vi "Get Speed For Shooting.vi"() -> (3 "Speed":dbl)   [LabVIEW 2016]
uses:
  Shared/Shooter Speed Type Def.ctl
  <vilib>/Rock Robotics/Network Tables/NT Read Boolean.vi
  Implementation/Ball Shooter Global.vi
  Framework/Robot Global Data.vi
  <vilib>/Analysis/NI_AALPro.lvlib
panel:
  in  "ClockWork":T1[](array[typedef])=[{"Distance"=8.5, "Speed"=5.4}, {"Distance"=10.9, "Speed"=6.3}, {"Distance"=8.1, "Speed"=5.1}]
  in  "Debug":bool
  out "XY Graph":cluster{dbl[], dbl[]}[](graph)
  in  "Veronica":T1[](array[typedef])=[{"Distance"=4.5, "Speed"=4.5}, {"Distance"=6.0, "Speed"=5.5}, {"Distance"=5.7, "Speed"=5.1}]
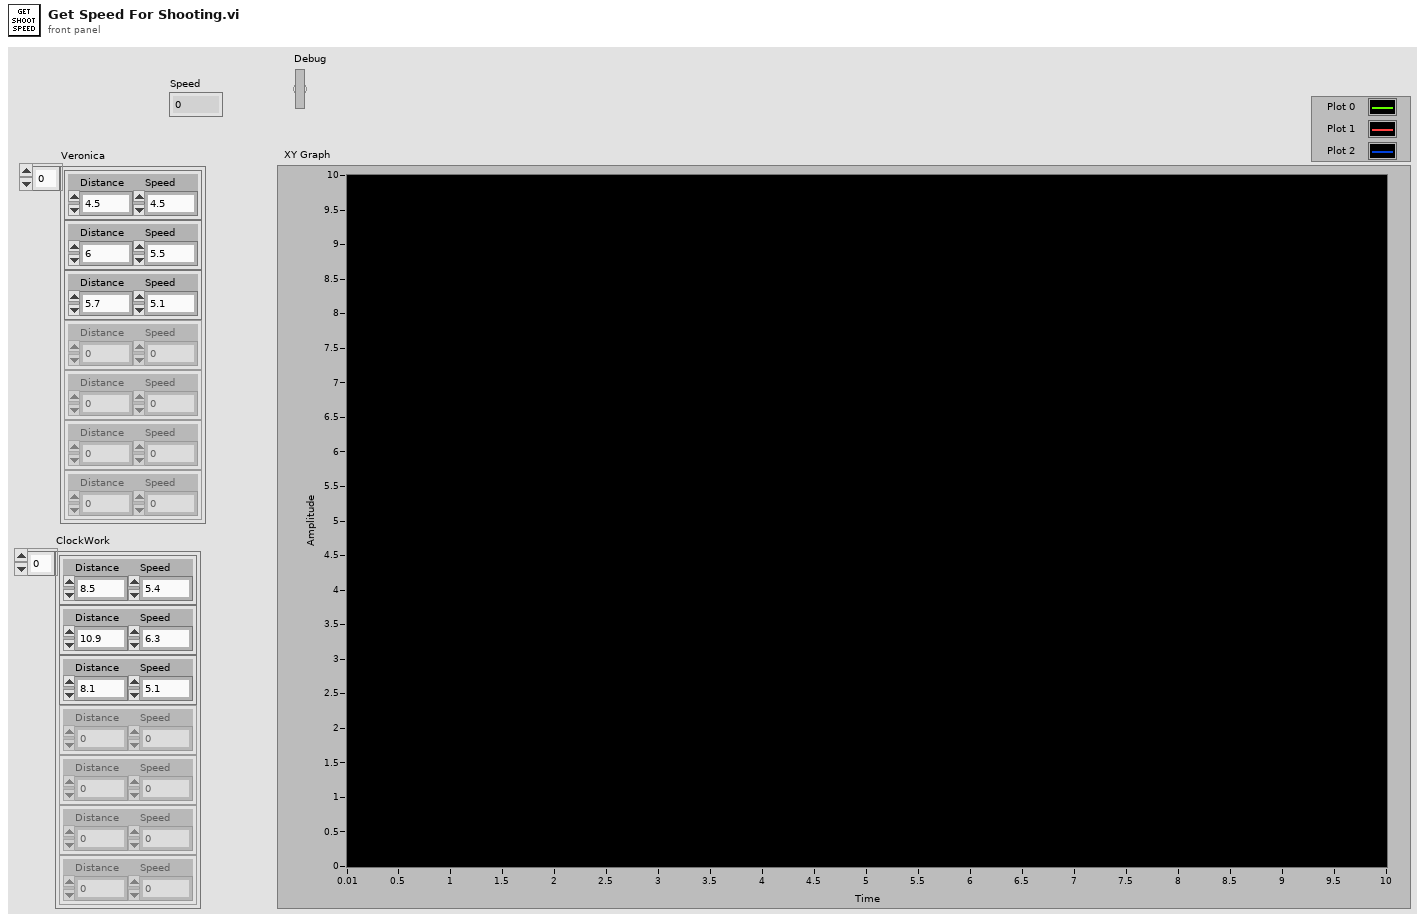
[diagram p1: front panel]
types:
  T1 = typedef "Shooter Speed Type Def.ctl" = cluster{"Distance":dbl, "Speed":dbl}
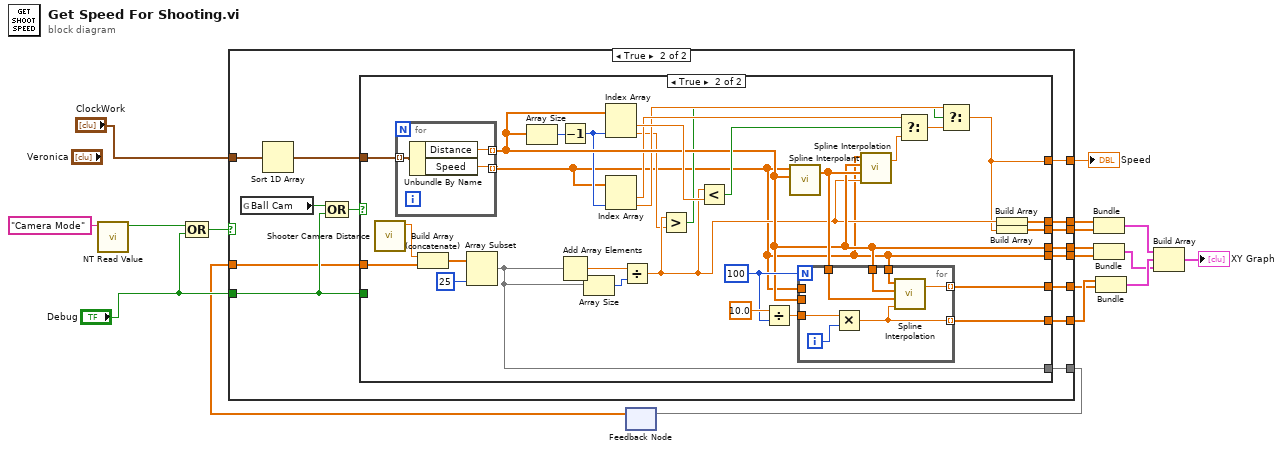
[diagram p0: block diagram]
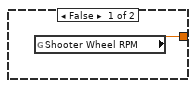
[diagram p2: hidden frame]
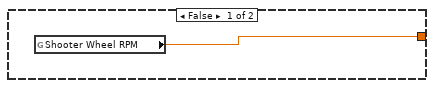
[diagram p3: hidden frame]
diagram:
  n1 = call-poly <vilib>:"NT Read Value.vi"("Name"="Camera Mode") -> ("Boolean"=w17:bool)  [unwired: 9 in, 1 out]
  n2 = Compound Arithmetic op=OR(w17, "Debug") -> (w13:bool)
  n3 = feedback #1() -> (w2:dbl[])  [unwired: 1 in]
  n4 = case shown="True" w13 {
    tunnel: "ClockWork" -> [_ w24]
    tunnel: [w19 w33] -> w16
    tunnel: [_ w32] -> w15
    tunnel: [_ w31] -> w14
    tunnel: "Debug" -> [_ w28]
    tunnel: [_ w27] -> w8
    tunnel: [_ w26] -> w11
    tunnel: [_ w25] -> w10
    tunnel: [_ w22] -> w7
    tunnel: [_ w21] -> w3
    tunnel: w2 -> [_ w20]
    frame False {
      n5 = global read "Ball Shooter Global.vi" "Shooter Wheel RPM"() -> (w19:dbl)
    }
    frame True {
      n6 = global read "Robot Global Data.vi" "Ball Cam"() -> (w30:bool)
      n7 = Sort 1D Array(array=w24) -> (sorted array=w23:T1[])
      n8 = Compound Arithmetic op=OR(w30, w28) -> (w29:bool)
      n9 = case shown="True" w29 {
        tunnel: [w34 w37] -> w33
        tunnel: w23 -> [_ w64]
        tunnel: [_ w45] -> w32
        tunnel: [_ w35] -> w31
        tunnel: w28 -> [_ _]
        tunnel: [_ w63] -> w27
        tunnel: [_ w62] -> w26
        tunnel: [_ w61] -> w25
        tunnel: [_ w56] -> w22
        tunnel: [_ w51] -> w21
        tunnel: w20 -> [_ w50]
        frame False {
          n10 = global read "Ball Shooter Global.vi" "Shooter Wheel RPM"() -> (w34:dbl)
        }
        frame True {
          w59 = 100
          n11 = call "Shooter Camera Distance.vi"() -> ("Distance (ft)"=w49:dbl)  [unwired: 9 in, 2 out]
          n12 = for {
            tunnel: w64 -> [w74] mode=indexing
            tunnel: [w73] -> w45 mode=indexing
            tunnel: [w72] -> w35 mode=indexing
            n13 = Unbundle By Name(w74) -> ("Distance"=w73:dbl, "Speed"=w72:dbl)
          }
          n14 = Build Array (concatenate)(w49, w50) -> (w55:dbl[])
          n15 = Array Subset(array=w55, length=25) -> (w51:dbl[])  [unwired: 1 in]
          n16 = Array Size(array=w45) -> (size(s)=w44:i32)
          n17 = Decrement(x=w44) -> (x-1=w36:i32)
          n18 = Add Array Elements(numeric array=w51) -> (sum=w54:dbl)
          n19 = Array Size(array=w51) -> (size(s)=w53:i32)
          n20 = Index Array(array=w45, index #2=w36) -> (element #1=w48:dbl, element #2=w39:dbl)  [unwired: 1 in]
          n21 = Index Array(array=w35, index #2=w36) -> (element #1=w43:dbl, element #2=w41:dbl)  [unwired: 1 in]
          n22 = Divide(x=w54, y=w53) -> (x/y=w40:dbl)
          n23 = Greater?(x=w40, y=w39) -> (0:w38:bool)
          n24 = Less?(x=w40, y=w48) -> (x < y?=w46:bool)
          n25 = Divide(x=10.0, y=w59) -> (x/y=w58:dbl)
          n26 = call <vilib>:"Spline Interpolant.vi"("X"=w45, "Y"=w35) -> ("Interpolant"=w57:dbl[])  [unwired: 2 in, 1 out]
          n27 = for {
            N: w59 -> [_]
            tunnel: w35 -> [_]
            tunnel: w45 -> [_]
            tunnel: w58 -> [w70]
            tunnel: [w66] -> w63 mode=indexing
            tunnel: w35 -> [w69]
            tunnel: w45 -> [w68]
            tunnel: w57 -> [w67]
            tunnel: [w65] -> w56 mode=indexing
            i -> [w71]
            n28 = Multiply(x=w70, y=w71) -> (x*y=w66:dbl)
            n29 = call <vilib>:"Spline Interpolation.vi"("x value"=w66, "Interpolant"=w67, "X"=w68, "Y"=w69) -> ("interpolation value"=w65:dbl)  [unwired: 1 out]
          }
          n30 = call <vilib>:"Spline Interpolation.vi"("x value"=w40, "Interpolant"=w57, "X"=w45, "Y"=w35) -> ("interpolation value"=w47:dbl)  [unwired: 1 out]
          n31 = Select(t=w43, s=w46, f=w47) -> (s? t:f=w42:dbl)
          n32 = Select(t=w41, s=w38, f=w42) -> (s? t:f=w37:dbl)
          n33 = Build Array(w40) -> (w62:dbl[])
          n34 = Build Array(w37) -> (w61:dbl[])
        }
      }
    }
  }
  "Speed" <- w16
  n35 = feedback-in #1(w3) -> ()
  n36 = Bundle(w11, w10) -> (w6:cluster{dbl[], dbl[]})  [unwired: 1 in]
  n37 = Bundle(w15, w14) -> (w4:cluster{dbl[], dbl[]})  [unwired: 1 in]
  n38 = Bundle(w8, w7) -> (w5:cluster{dbl[], dbl[]})  [unwired: 1 in]
  n39 = Build Array(w6, w5, w4) -> (→"XY Graph":cluster{dbl[], dbl[]}[])
